vi "ATF-Pump-Drive_Read_A.vi"(8 "error in":errorcluster, 11 "Data FIFO Ref":T1) -> (0 "error out":errorcluster)   [LabVIEW 2022 SP3]
uses:
  RT Controls/ATF-Pump-Data FIFO.ctl
  RT Support/ATF-Pump-RT_Global_R.vi
panel:
  in  "TCP_Port_Bottom":u16=3000
  in  "TCP_Port_Top":u16=2000
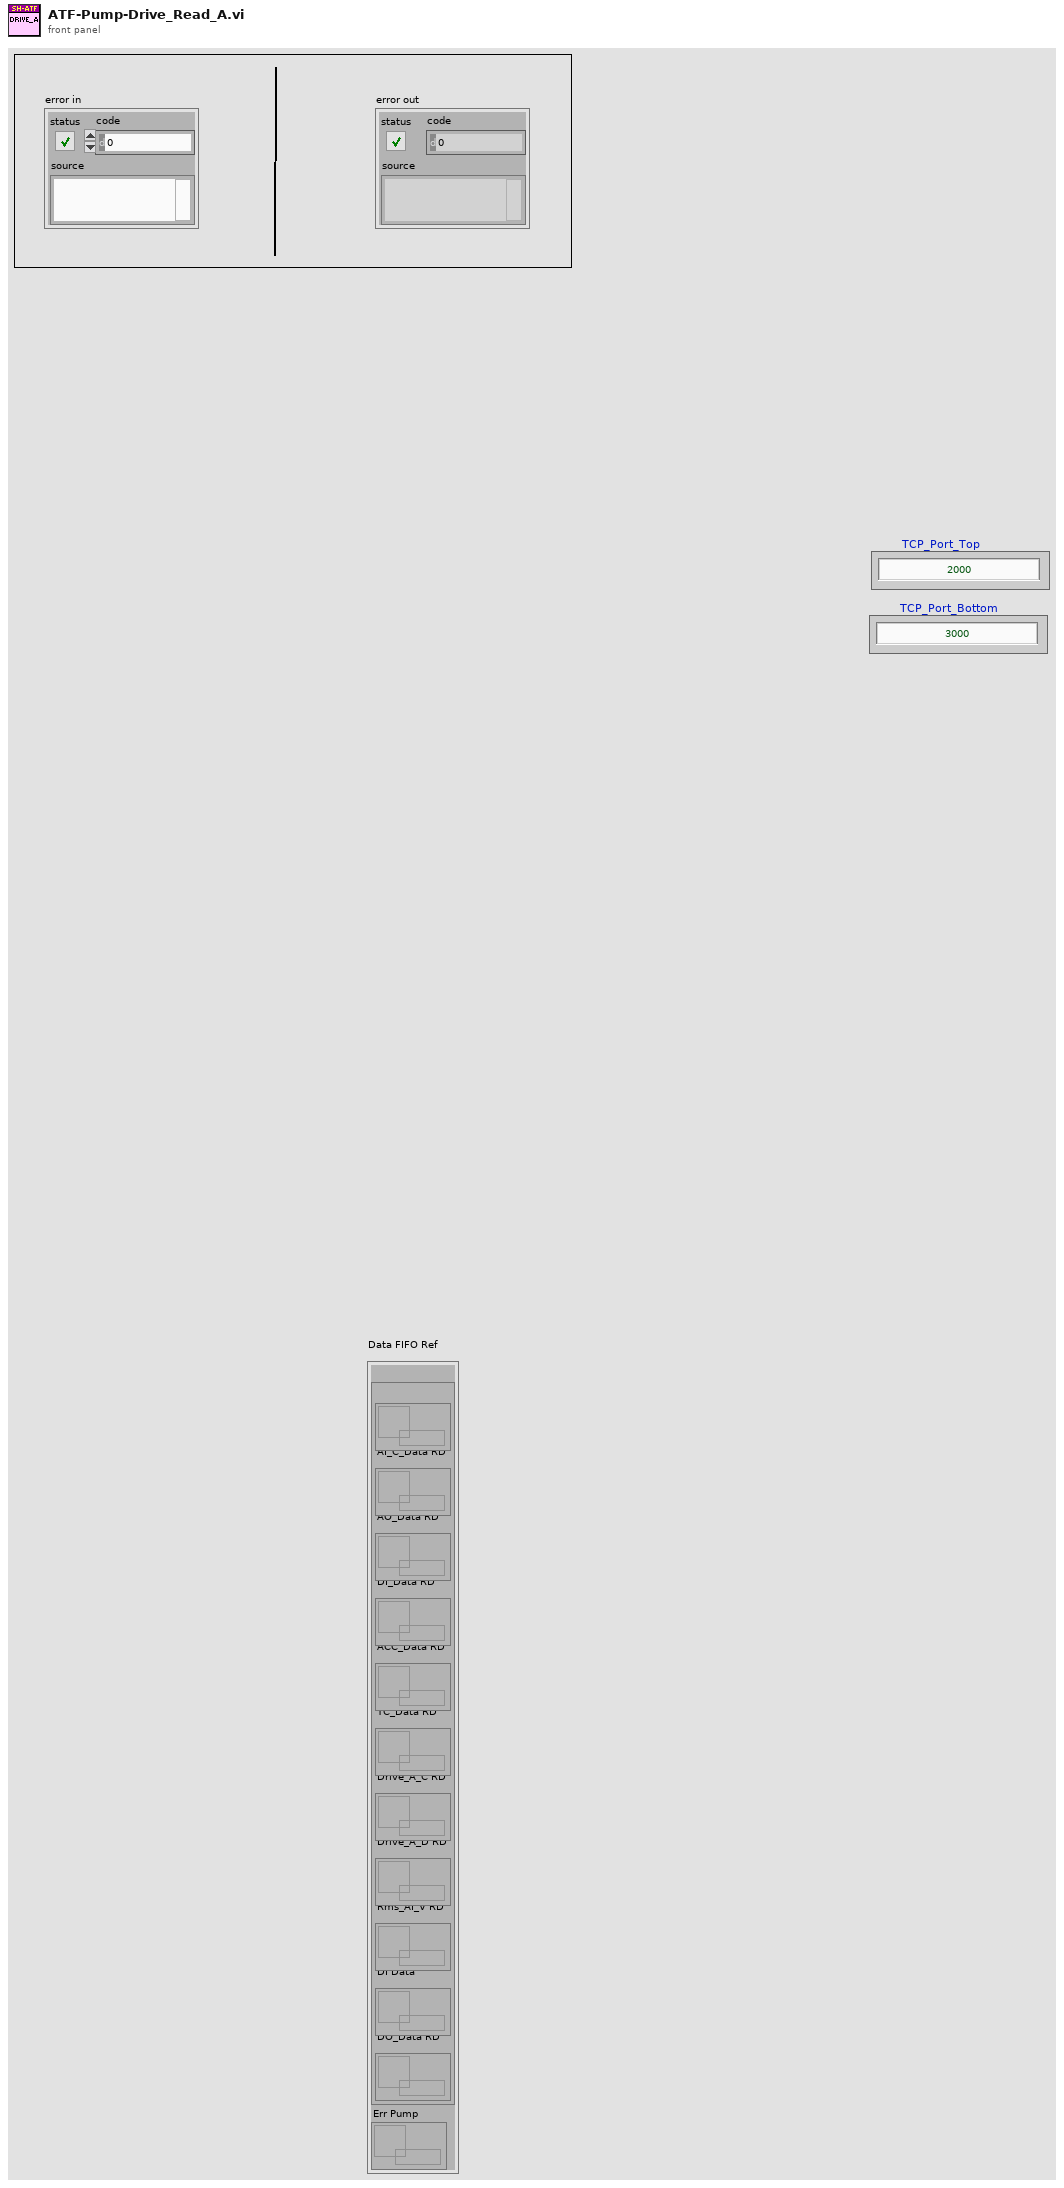
[diagram p1: front panel]
types:
  T1 = typedef "ATF-Pump-Data FIFO.ctl" = cluster{"RD":cluster{"AI_V_Data RD":refnum<queue>, "AI_C_Data RD":refnum<queue>, "AO_Data RD":refnum<queue>, "DI_Data RD":refnum<queue>, "ACC_Data RD":refnum<queue>, "TC_Data RD":refnum<queue>, "Drive_A_C RD":refnum<queue>, "Drive_A_D RD":refnum<queue>, "Rms_AI_V RD":refnum<queue>, "DI Data":refnum<queue>, "DO_Data RD":refnum<queue>}, "Err Pump":refnum<queue>}
  T2 = cluster{"En_Drive_A":bool, "En_Drive_L":bool, "Exit_Drive_A":bool, "Exit_Drive_L":bool}
  T3 = enum16{"AI C", "AI V", "AO", "DI", "DO", "TC", "ACC", "RT PMP", "DR A"}
  T4 = enum16{"Init", "Read 'All'", "Read 'n'", "Read '1'", "Write '1'", "Write 'n'", "Write 'All'"}
  T5 = cluster{"Start DAQ":bool, "Stop DAQ":bool, "RT Stop":bool, "RT Exit":bool, "Start Seq":bool}
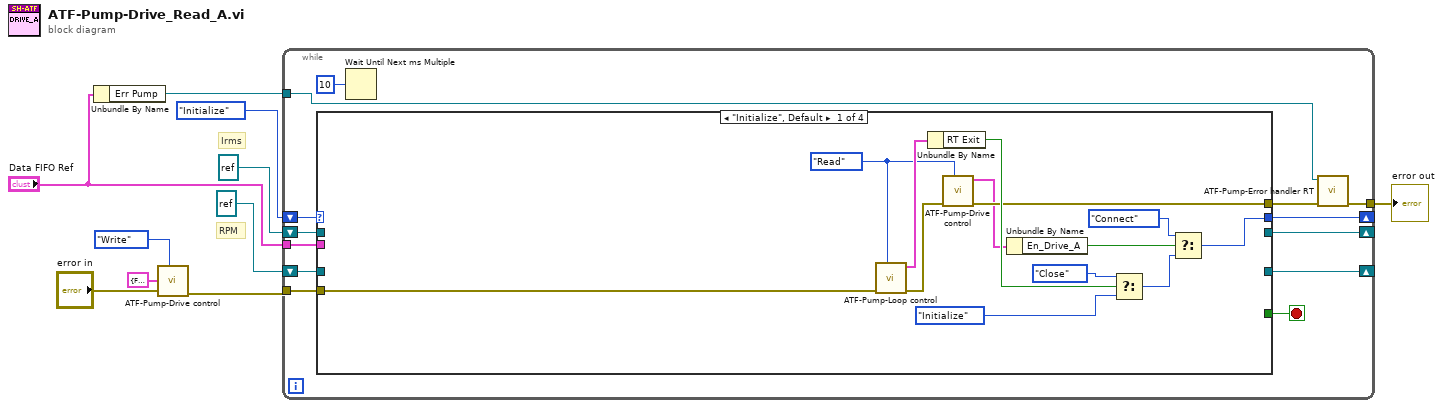
[diagram p0: block diagram]
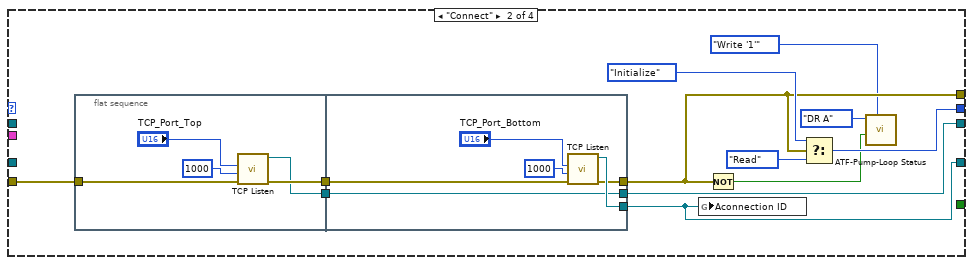
[diagram p2: hidden frame]
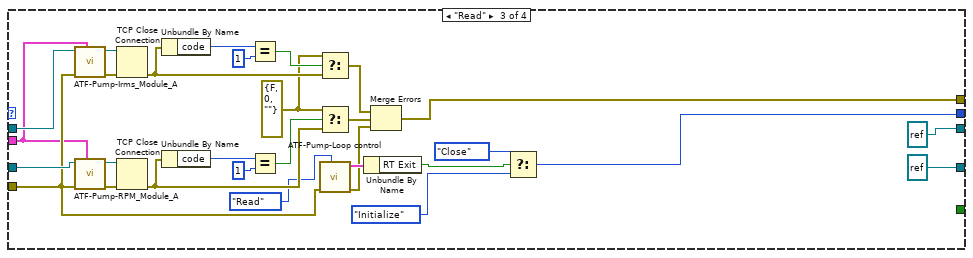
[diagram p3: hidden frame]
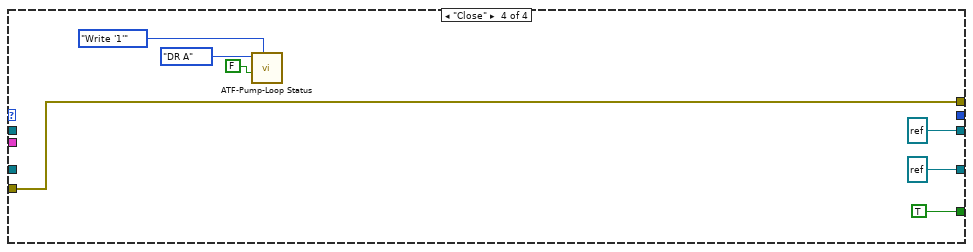
[diagram p4: hidden frame]
diagram:
  # "RPM"
  # "Irms"
  n1 = Unbundle By Name("Data FIFO Ref") -> ("Err Pump"=w5:refnum<queue>)
  n2 = call "ATF-Pump-Drive control.vi"("Action"=enum16{"Init", "Write", "Read"}."Write", "error in"="error in", "Loop Control In"=T2 {"En_Drive_A"=FALSE, "En_Drive_L"=FALSE, "Exit_Drive_A"=FALSE, "Exit_Drive_L"=FALSE}) -> ("error Out"=w3:errorcluster)  [unwired: 7 in, 1 out]
  n3 = while {
    shift-right: [w22] -> _
    shift-left: enum16{"Initialize", "Connect", "Read", "Close"}."Initialize" -> [w23]
    tunnel: w3 -> [w21]
    tunnel: [w13] -> w9
    shift-right: [w20] -> _
    shift-left: refnum<k5> refnum ("connection ID") -> [w18]
    shift-right: [w19] -> _
    shift-left: refnum<k5> refnum ("connection ID") -> [w17]
    tunnel: "Data FIFO Ref" -> [w15]
    tunnel: w5 -> [w12]
    stop <- w16 stop-if-true
    n4 = case shown="\"Initialize\", Default" w23 {
      tunnel: [w36 w42 w86 _] -> w22
      tunnel: w21 -> [w29 w46 w61 w92]
      tunnel: [w28 w41 w74 w92] -> w14
      tunnel: [_ w45 refnum<k5> refnum ("TCP Network Connection out") refnum<k5> refnum ("TCP Network Connection out")] -> w20
      tunnel: [_ w40 refnum<k5> refnum ("TCP Network Connection out") refnum<k5> refnum ("TCP Network Connection out")] -> w19
      tunnel: w18 -> [_ _ w69 _]
      tunnel: w17 -> [_ _ w68 _]
      tunnel: [_ _ _ TRUE] -> w16
      tunnel: w15 -> [_ _ w60 _]
      frame "Initialize", Default {
        w24 = enum16{"Init", "Write", "Read"}."Read" ("Action")
        n5 = call "ATF-Pump-Loop control.vi"("Action"=w24, "error in (no error)"=w29) -> ("error Out"=w27:errorcluster, "Loop Control out"=w31:T5)  [unwired: 8 in]
        n6 = Unbundle By Name(w31) -> ("RT Exit"=w30:bool)
        n7 = call "ATF-Pump-Drive control.vi"("Action"=w24, "error in"=w27) -> ("error Out"=w28:errorcluster, "Loop Control Out"=w26:T2)  [unwired: 8 in]
        n8 = Unbundle By Name(w26) -> ("En_Drive_A"=w25:bool)
        n9 = Select(t=enum16{"Initialize", "Connect", "Read", "Close"}."Close", s=w30, f=enum16{"Initialize", "Connect", "Read", "Close"}."Initialize") -> (s? t:f=w32:enum16{"Initialize", "Connect", "Read", "Close"})
        n10 = Select(t=enum16{"Initialize", "Connect", "Read", "Close"}."Connect", s=w25, f=w32) -> (s? t:f=w36:enum16{"Initialize", "Connect", "Read", "Close"})
      }
      frame "Connect" {
        n11 = flat-sequence {
          tunnel: w46 -> [w51]
          tunnel: [w50] -> w48
          tunnel: [w49] -> w47
          tunnel: [w59] -> w40
          tunnel: w48 -> [w55]
          tunnel: w47 -> [w58]
          tunnel: [w58] -> w45
          tunnel: [w54] -> w41
          frame #0 {
            n12 = call <vilib>:"TCP Listen.vi"("error in (no error)"=w51, "timeout ms (wait forever: -1)"=1000, "port"="TCP_Port_Top") -> ("error out"=w50:errorcluster, "connection ID"=w49:refnum<k5>)  [unwired: 4 in, 3 out]
          }
          frame #1 {
            n13 = call <vilib>:"TCP Listen.vi"("error in (no error)"=w55, "timeout ms (wait forever: -1)"=1000, "port"="TCP_Port_Bottom") -> ("error out"=w54:errorcluster, "connection ID"=w59:refnum<k5>)  [unwired: 4 in, 3 out]
          }
        }
        n14 = global write "ATF-Pump-RT_Global_R.vi" "Aconnection ID"(w40) -> ()
        n15 = Not(x=w41) -> (.not. x?=w38:bool)
        n16 = Select(t=enum16{"Initialize", "Connect", "Read", "Close"}."Initialize", s=w41, f=enum16{"Initialize", "Connect", "Read", "Close"}."Read") -> (s? t:f=w42:enum16{"Initialize", "Connect", "Read", "Close"})
        n17 = call "ATF-Pump-Loop Status.vi"("Option"=T4."Write '1'", "Status"=w38, "Loop"=T3."DR A") -> ()  [unwired: 6 in, 3 out]
      }
      frame "Read" {
        w77 = errorcluster {"status"=FALSE, "code"=0, "source"=""} ("error constant")
        n18 = call "ATF-Pump-Irms_Module_A.vi"("Data FIFO Ref"=w60, "error in"=w61, "TCP Network Connection in"=w69) -> ("error out"=w70:errorcluster, "TCP Network Connection out"=w71:refnum<k5>)  [unwired: 7 in]
        n19 = call "ATF-Pump-RPM_Module_A.vi"("Data FIFO Ref"=w60, "error in (no error)"=w61, "TCP Network Connection in"=w68) -> ("error out"=w66:errorcluster, "TCP Network Connection out"=w67:refnum<k5>)  [unwired: 7 in]
        n20 = TCP Close Connection(connection ID=w71, error in (no error)=w70) -> (error out=w81:errorcluster)  [unwired: 1 in, 1 out]
        n21 = TCP Close Connection(connection ID=w67, error in (no error)=w66) -> (error out=w80:errorcluster)  [unwired: 1 in, 1 out]
        n22 = Unbundle By Name(w81) -> ("code"=w85:i32)
        n23 = Unbundle By Name(w80) -> ("code"=w84:i32)
        n24 = Equal?(x=w85, y=1) -> (x = y?=w82:bool)
        n25 = Equal?(x=w84, y=1) -> (x = y?=w83:bool)
        n26 = Select(t=w77, s=w82, f=w81) -> (s? t:f=w79:errorcluster)
        n27 = Select(t=w77, s=w83, f=w80) -> (s? t:f=w78:errorcluster)
        n28 = call "ATF-Pump-Loop control.vi"("Action"=enum16{"Init", "Write", "Read"}."Read", "error in (no error)"=w61) -> ("error Out"=w62:errorcluster, "Loop Control out"=w65:T5)  [unwired: 8 in]
        n29 = Unbundle By Name(w65) -> ("RT Exit"=w64:bool)
        n30 = Merge Errors(w79, w78, w62) -> (w74:errorcluster)
        n31 = Select(t=enum16{"Initialize", "Connect", "Read", "Close"}."Close", s=w64, f=enum16{"Initialize", "Connect", "Read", "Close"}."Initialize") -> (s? t:f=w86:enum16{"Initialize", "Connect", "Read", "Close"})
      }
      frame "Close" {
        n32 = call "ATF-Pump-Loop Status.vi"("Option"=T4."Write '1'", "Status"=FALSE, "Loop"=T3."DR A") -> ()  [unwired: 6 in, 3 out]
      }
    }
    n33 = Wait Until Next ms Multiple(millisecond multiple=u32 10) -> ()  [unwired: 1 out]
    n34 = call "ATF-Pump-Error handler RT.vi"("error in"=w14, "Message Queue"=w12) -> ("error out"=w13:errorcluster)  [unwired: 8 in, 1 out]
  }
  "error out" <- w9
